vi "Create Privite Events.vi"(8 "error in (no error)":errorcluster, 11 "XY Stage Process in":refnum<class "XY Stage Process.lvclass">) -> (0 "error out":errorcluster, 3 "XY Stage Process out":refnum<class "XY Stage Process.lvclass">)   [LabVIEW 2022 SP3, in "XY Stage Process.lvlib" / "XY Stage Process.lvclass"]
uses:
  XY Stage Process.lvclass
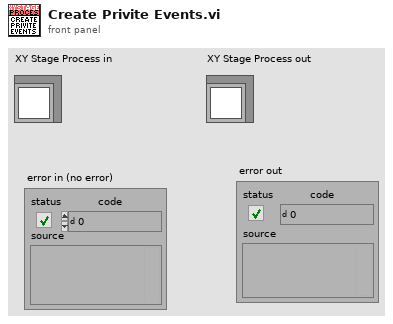
[diagram p1: front panel]
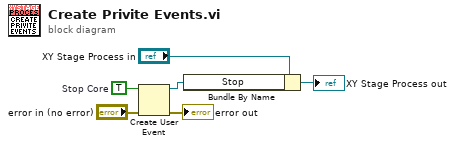
[diagram p0: block diagram]
diagram:
  w4 = TRUE  # Stop Core
  n1 = Create User Event(user event datatype=w4, error in="error in (no error)") -> (user event=w6:refnum<user-event>, error out=→"error out":errorcluster)
  n2 = Bundle By Name(cluster="XY Stage Process in", "Stop"=w6) -> (→"XY Stage Process out":refnum<class "XY Stage Process.lvclass">)
